vi "Serial float Read from ATMega32.vi"() -> ()   [LabVIEW 2016]
uses:
  <vilib>/Instr/_visa.llb/VISA Configure Serial Port (Instr).vi
panel:
  in  "stop 2":bool
  out "Waveform Chart":dbl(graph)
  out "return count":u32
  out "?":u8[](array[numeric])
  out "Array":dbl[](array[numeric])
  out "Numeric":fxp<+,32,32>
  in  "stop":bool
  in  "flow control (0:none)":u16(ring) items=["None", "XON/XOFF", "RTS/CTS", "XON/XOFF & RTS/CTS", "DTR/DSR", "XON/XOFF & DTR/DSR"]
  in  "VISA resource name":refnum<visa-resource-name>
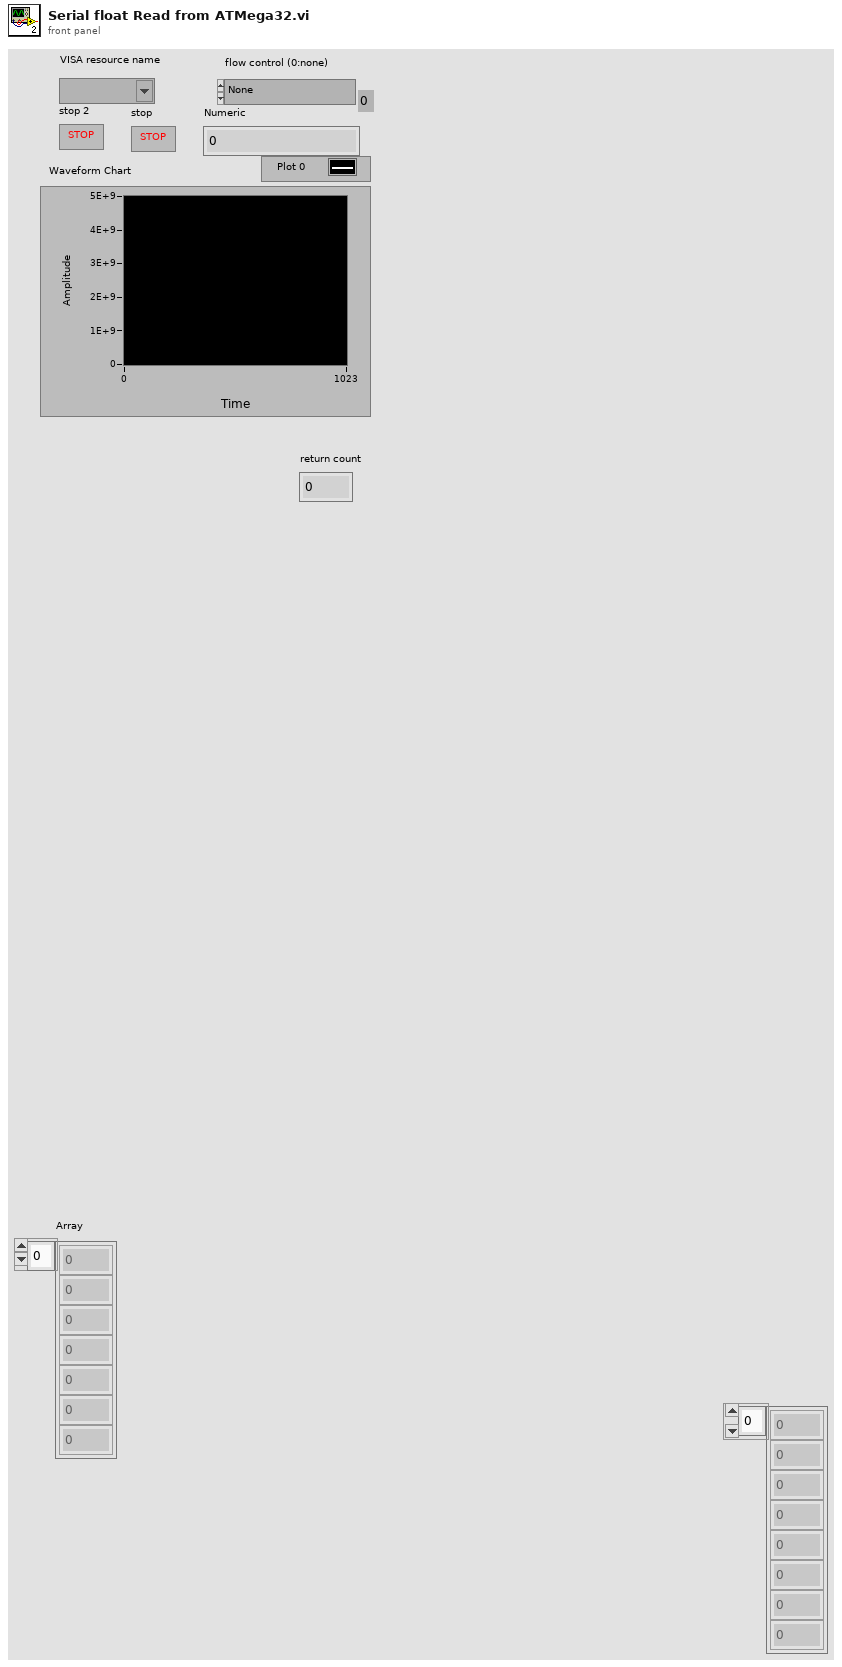
[diagram p1: front panel]
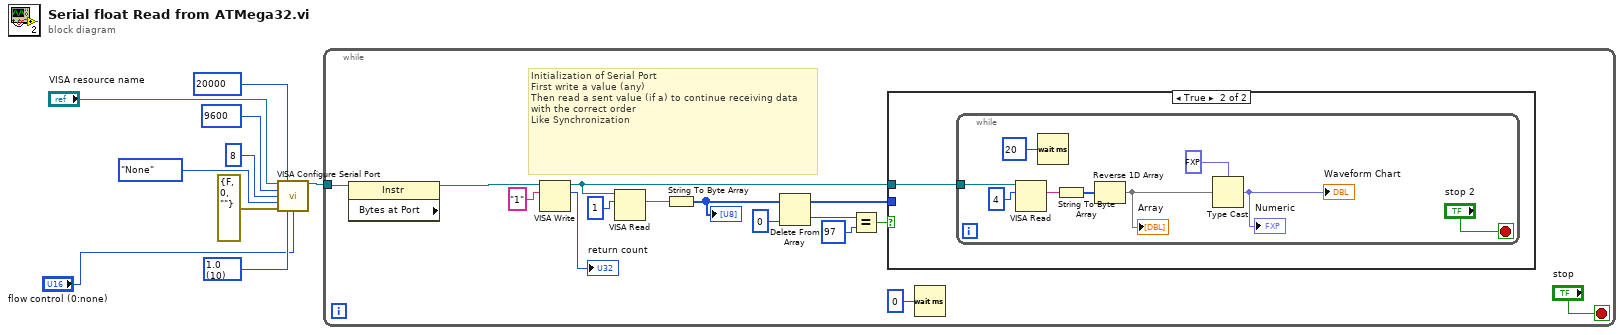
[diagram p0: block diagram]
diagram:
  w4 = u16 10 items=["1.0"=10, "1.5"=15, "2.0"=20] ("stop bits (10: 1 bit)")
  n1 = call-poly "VISA Configure Serial Port"("VISA resource name"="VISA resource name", "timeout (10sec)"=u32 20000, "baud rate (9600)"=u32 9600, "data bits (8)"=u16 8, "parity (0:none)"=enum16{"None", "Odd", "Even", "Mark", "Space"}."None", "error in (no error)"=errorcluster {"status"=FALSE, "code"=0, "source"=""}, "stop bits (10: 1 bit)"=w4, "flow control (0:none)"="flow control (0:none)") -> ("VISA resource name out"=w2:refnum<visa-resource-name>)  [unwired: 6 in, 1 out]
  n2 = while {
    tunnel: w2 -> [w24]
    stop <- "stop" stop-if-true
    # "Initialization of Serial Port\nFirst write a value (any)\nThen read a sent value (if a) to continue receiving data with the correct order\nLike Synchronization"
    n3 = property class="Instr" props=["Bytes at Port"](reference=w24) -> (reference out=w11:refnum<visa-resource-name>)  [unwired: 1 in, 2 out]
    n4 = VISA Write(VISA resource name=w11, write buffer="1") -> (VISA resource name out=w10:refnum<visa-resource-name>, return count=→"return count":u32)  [unwired: 1 in, 1 out]
    n5 = VISA Read(VISA resource name=w10, byte count=1) -> (read buffer=w18:string)  [unwired: 1 in, 3 out]
    n6 = String To Byte Array(string=w18) -> (unsigned byte array=w19:u8[])
    "?" <- w19
    n7 = Delete From Array(array=w19, index=0) -> (deleted portion=w15:u8, array with subset deleted=w17:u8[])  [unwired: 1 in]
    n8 = Equal?(x=w15, y=u8 97) -> (x = y?=w16:bool)
    n9 = case shown="True" w16 {
      tunnel: w17 -> [_ _]
      tunnel: w10 -> [_ w25]
      frame False {
      }
      frame True {
        n10 = while {
          tunnel: w25 -> [w31]
          stop <- "stop 2" stop-if-true
          n11 = VISA Read(VISA resource name=w31, byte count=u32 4) -> (read buffer=w32:string)  [unwired: 1 in, 3 out]
          n12 = Wait (ms)(milliseconds to wait=u32 20) -> ()  [unwired: 1 out]
          n13 = String To Byte Array(string=w32) -> (unsigned byte array=w29:u8[])
          n14 = Reverse 1D Array(array=w29) -> (reversed array=w33:u8[])
          "Array" <- w33
          n15 = Type Cast(type=fxp<+,32,32> 0.0, x=w33) -> (*(type *) &x=→"Numeric" →"Waveform Chart":fxp<+,32,32>)
        }
      }
    }
    n16 = Wait (ms)(milliseconds to wait=u32 0) -> ()  [unwired: 1 out]
  }
